vi "Dense - Scale Problem Linear.vi"(8 "error in (no error)":errorcluster, 9 "Y Scaling limits":cluster{"Y lower":dbl, "Y upper":dbl}={"Y lower"=nan, "Y upper"=nan}, 10 "X Scaling limits":cluster{"X lower":dbl, "X upper":dbl}={"X lower"=0.0, "X upper"=1.0}, 11 "Problem":T1) -> (0 "error out":errorcluster, 1 "ymaxmin":cluster{"ymax":dbl, "ymin":dbl}, 2 "xmaxmin":cluster{"min":dbl, "max":dbl}[](array[cluster]), 3 "Scaled problem":T1)   [LabVIEW 2015]
doc: "Scales the problem similarly to the svm-scale tool bundled with libsvm.\nAlways use the output from this VI to scale the test set instead of scaling individually.\n\nNote that dense and sparse xmaxmin are not compatible, as the 0th index is unused for sparse."
uses:
  LibSVM Dense/Wrapper API/Controls/svmdense_problem.ctl
  Controls/Statemachine_ScaleProblem.ctl
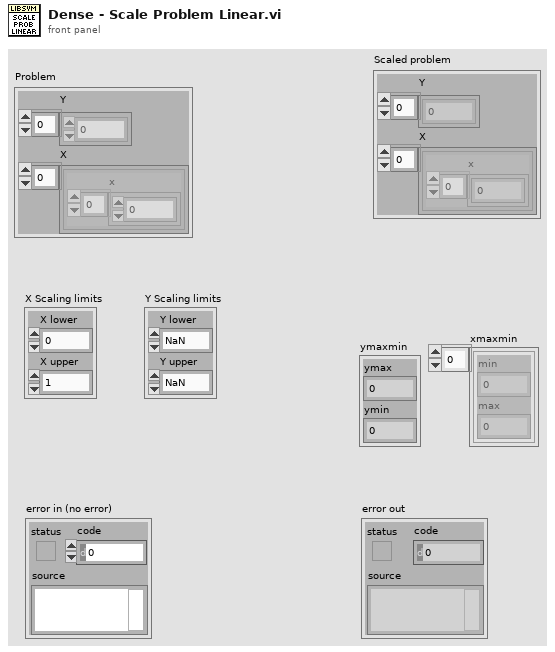
[diagram p1: front panel]
types:
  T1 = typedef "svmdense_problem.ctl" = cluster{"Y":dbl[], "X":cluster{"x":dbl[]}[]}
  T2 = typedef "Statemachine_ScaleProblem.ctl" = enum16{"Input verification: Limits", "Input verification: Ascending indices", "Find max/min index", "Find max/min features", "Scale", "Stop"}
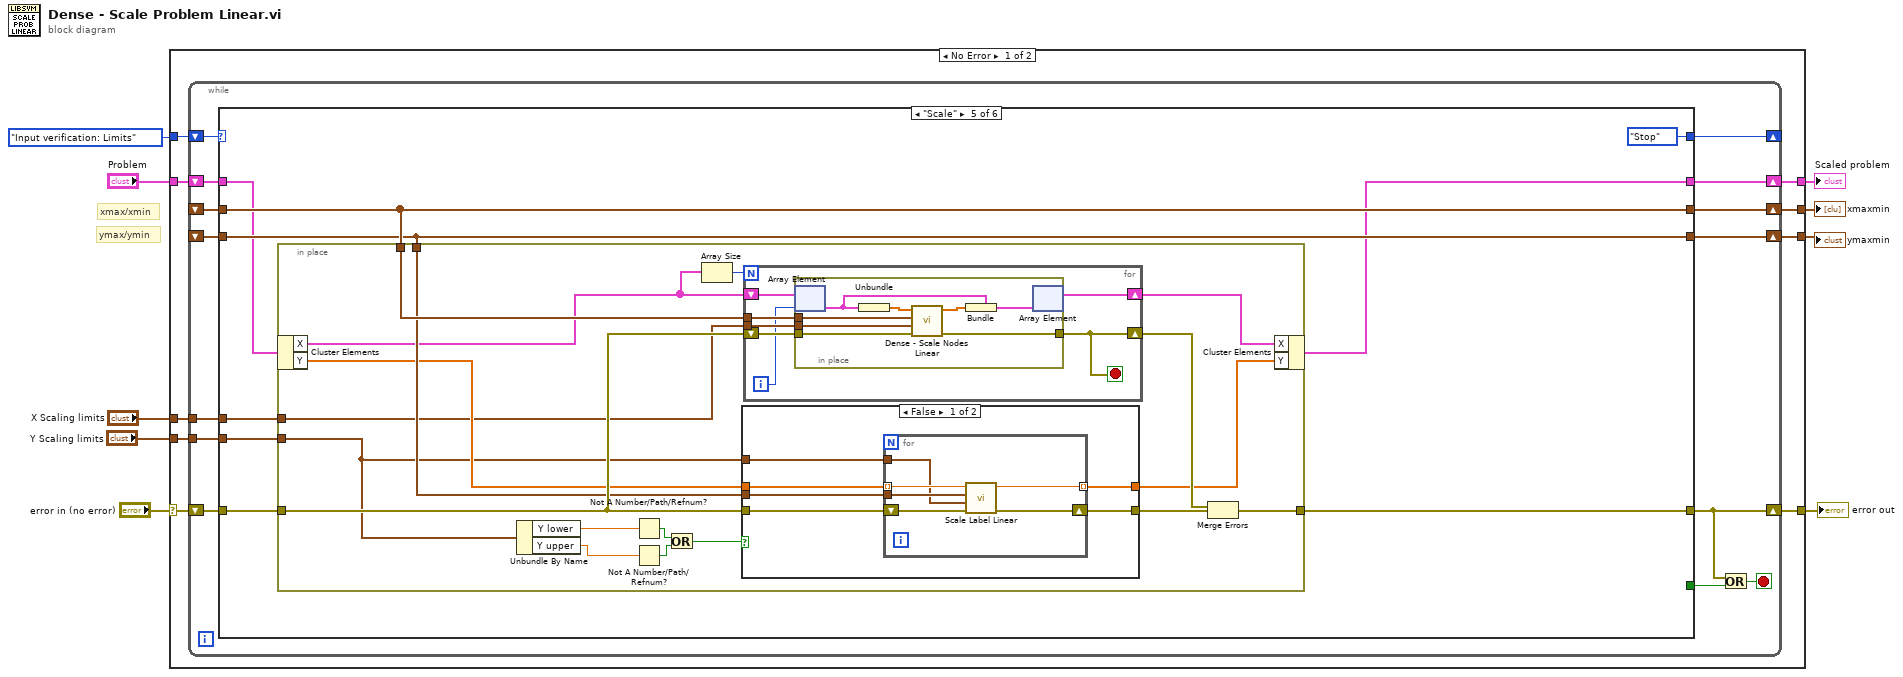
[diagram p0: block diagram]
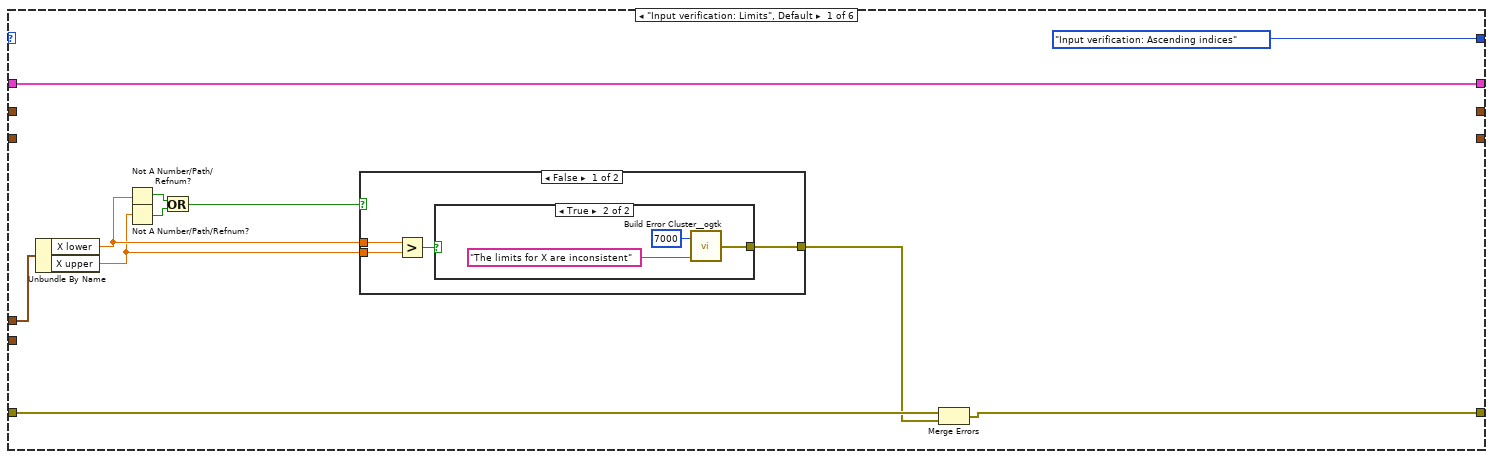
[diagram p2: hidden frame]
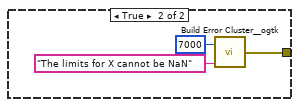
[diagram p4: hidden frame]
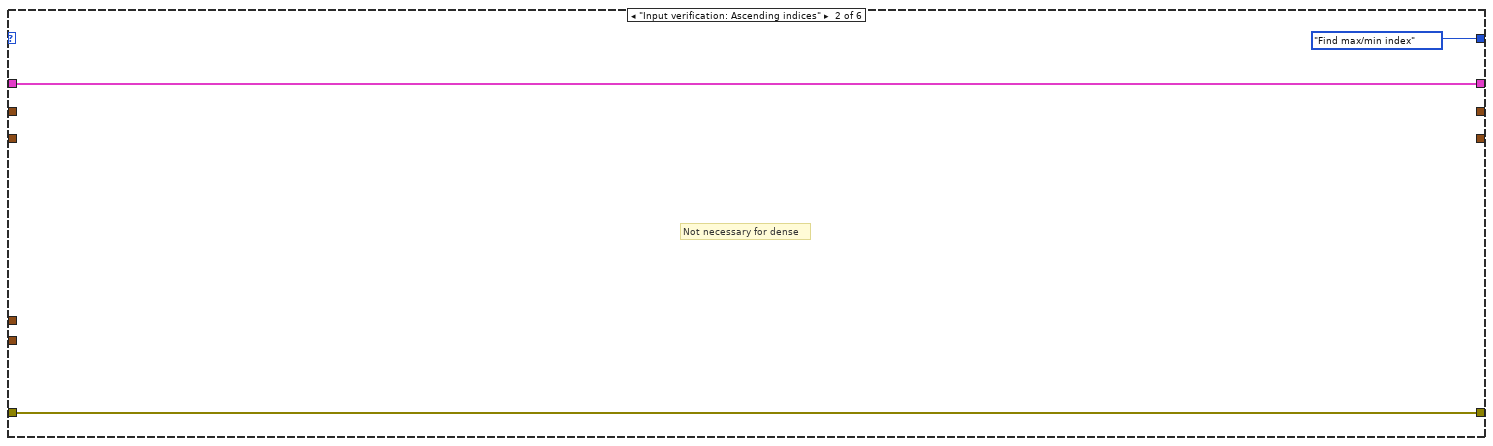
[diagram p5: hidden frame]
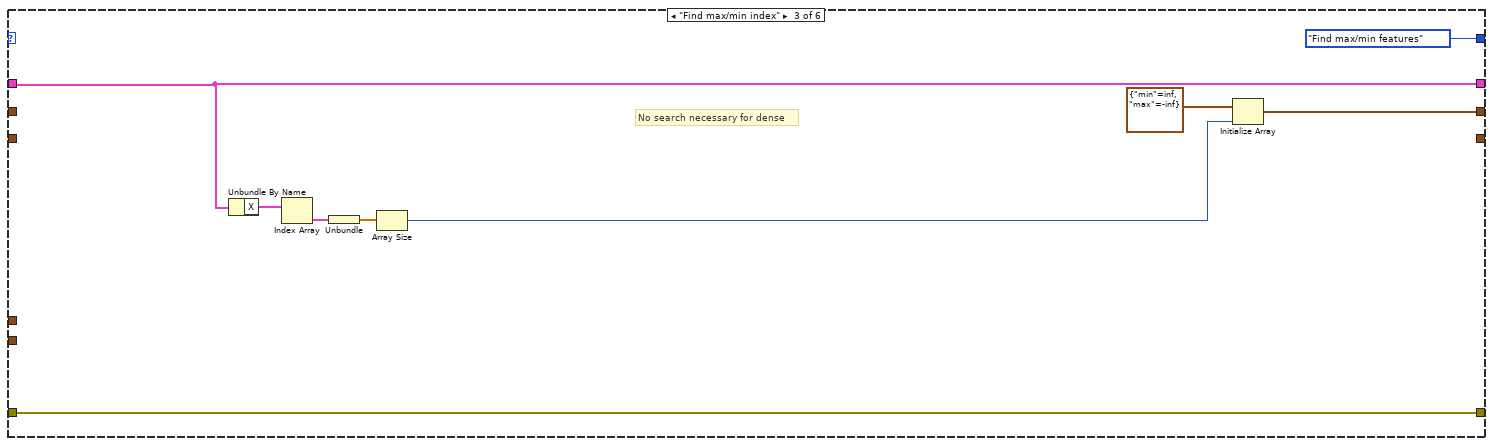
[diagram p6: hidden frame]
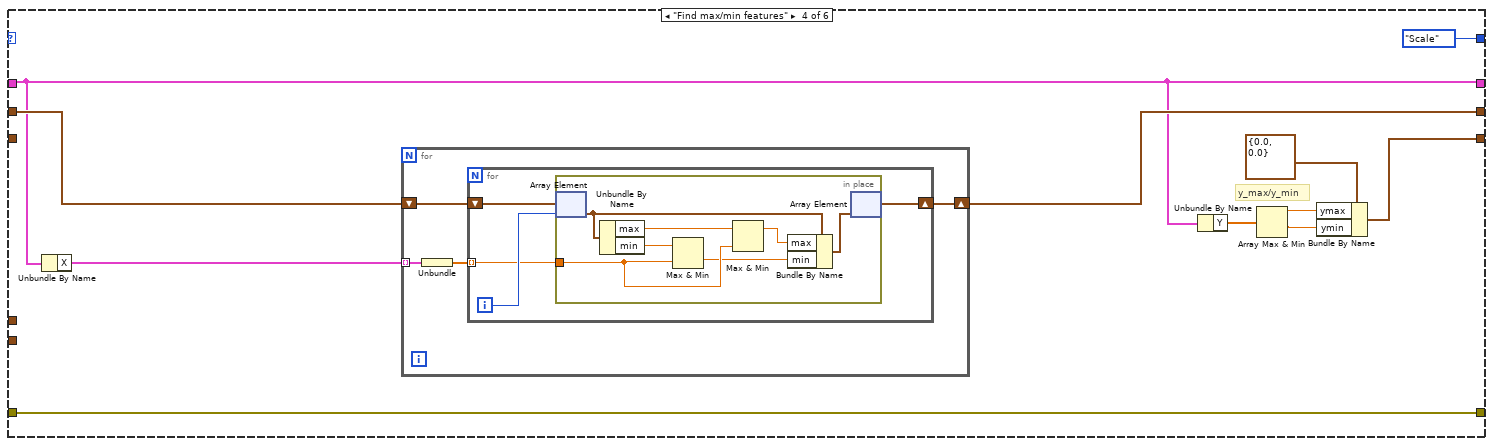
[diagram p7: hidden frame]
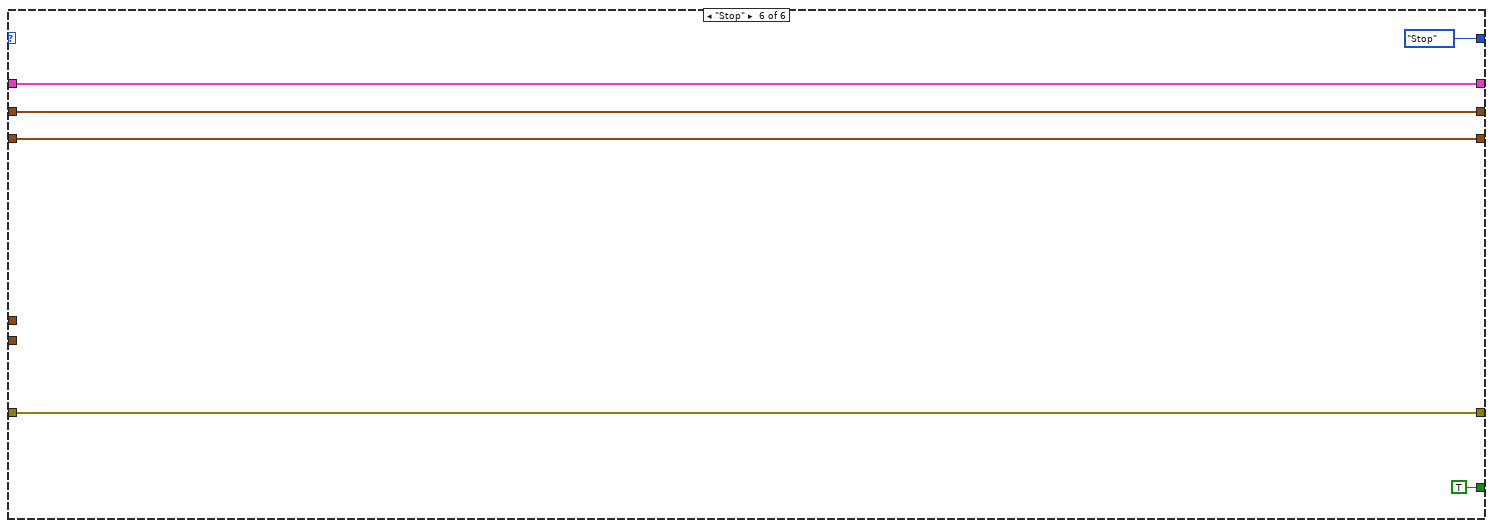
[diagram p9: hidden frame]
diagram:
  # "ymax/ymin"
  # "xmax/xmin"
  n1 = case shown="No Error" "error in (no error)" {
    selector: "error in (no error)" -> [w18 w154]
    tunnel: [w15 w154] -> w9
    tunnel: "Problem" -> [w11 _]
    tunnel: "X Scaling limits" -> [w16 _]
    tunnel: Statemachine_ScaleProblem."Input verification: Limits" ("Statemachine_ScaleProblem") -> [w17 _]
    tunnel: [w14 _] -> w4
    tunnel: [w13 _] -> w5
    tunnel: [w12 _] -> w2
    tunnel: "Y Scaling limits" -> [w10 _]
    frame No Error {
      n2 = while {
        shift-right: [w29] -> _
        shift-left: w17 -> [w32]
        tunnel: w16 -> [w31]
        shift-right: [w22] -> w15
        shift-left: w18 -> [w30]
        shift-right: [w28] -> w13
        shift-left: _ -> [w27]
        shift-right: [w26] -> w14
        shift-left: _ -> [w25]
        shift-right: [w24] -> w12
        shift-left: w11 -> [w23]
        tunnel: w10 -> [w19]
        stop <- w21 stop-if-true
        n3 = case shown="\"Scale\"" w32 {
          tunnel: w31 -> [w43 _ _ _ w99 _]
          tunnel: w30 -> [w37 w56 w57 w73 w98 w152]
          tunnel: [w35 w56 w57 w73 w97 w152] -> w22
          tunnel: [Statemachine_ScaleProblem."Input verification: Ascending indices" ("Statemachine_ScaleProblem") Statemachine_ScaleProblem."Find max/min index" ("Statemachine_ScaleProblem") Statemachine_ScaleProblem."Find max/min features" ("Statemachine_ScaleProblem") Statemachine_ScaleProblem."Scale" ("Statemachine_ScaleProblem") Statemachine_ScaleProblem."Stop" ("Statemachine_ScaleProblem") Statemachine_ScaleProblem."Stop" ("Statemachine_ScaleProblem")] -> w29
          tunnel: [_ _ w64 w74 w96 w151] -> w28
          tunnel: w27 -> [_ _ _ w75 w96 w151]
          tunnel: [_ _ _ w69 w95 w150] -> w26
          tunnel: w25 -> [_ _ _ _ w95 w150]
          tunnel: [w33 w54 w62 w67 w93 w149] -> w24
          tunnel: w23 -> [w33 w54 w62 w67 w94 w149]
          tunnel: [_ _ _ _ _ TRUE] -> w20
          tunnel: w19 -> [_ _ _ _ w92 _]
          frame "Input verification: Limits", Default {
            n4 = Unbundle By Name(w43) -> ("X lower"=w39:dbl, "X upper"=w38:dbl)
            n5 = Not A Number/Path/Refnum?(number/path/refnum=w39) -> (NaN/Path/Refnum?=w41:bool)
            n6 = Not A Number/Path/Refnum?(number/path/refnum=w38) -> (NaN/Path/Refnum?=w42:bool)
            n7 = Or(x=w41, y=w42) -> (x .or. y?=w40:bool)
            n8 = case shown="False" w40 {
              tunnel: w39 -> [w46 _]
              tunnel: w38 -> [w45 _]
              tunnel: [w44 w51] -> w36
              frame False {
                n9 = Greater?(x=w46, y=w45) -> (0:w47:bool)
                n10 = case shown="True" w47 {
                  tunnel: [_ w48] -> w44
                  frame False {
                  }
                  frame True {
                    n11 = call <userlib>:"Build Error Cluster__ogtk.vi"("String to Prepend to source (\"\")"="The limits for X are inconsistent" ("String to Prepend to source (\"\")"), "code"=7000) -> ("error out"=w48:errorcluster)
                  }
                }
              }
              frame True {
                n12 = call <userlib>:"Build Error Cluster__ogtk.vi"("String to Prepend to source (\"\")"="The limits for X cannot be NaN" ("String to Prepend to source (\"\")"), "code"=7000) -> ("error out"=w51:errorcluster)
              }
            }
            n13 = Merge Errors(w37, w36) -> (w35:errorcluster)
          }
          frame "Input verification: Ascending indices" {
            # "Not necessary for dense"
          }
          frame "Find max/min index" {
            # "No search necessary for dense"
            n14 = Unbundle By Name(w62) -> ("X"=w61:cluster{"x":dbl[]}[])
            n15 = Index Array(array=w61) -> (element=w60:cluster{"x":dbl[]})  [unwired: 1 in]
            n16 = Unbundle(w60) -> ("x"=w59:dbl[])
            n17 = Array Size(array=w59) -> (size(s)=w58:i32)
            n18 = Initialize Array(cluster{"min":dbl, "max":dbl} {"min"=inf, "max"=-inf}, w58) -> (w64:cluster{"min":dbl, "max":dbl}[])
          }
          frame "Find max/min features" {
            # "y_max/y_min"
            n19 = Unbundle By Name(w67) -> ("X"=w76:cluster{"x":dbl[]}[])
            n20 = for {
              tunnel: w76 -> [w80] mode=indexing
              shift-right: [w78] -> w74
              shift-left: w75 -> [w79]
              n21 = Unbundle(w80) -> ("x"=w77:dbl[])
              n22 = for {
                shift-right: [w83] -> w78
                shift-left: w79 -> [w84]
                tunnel: w77 -> [w81] mode=indexing
                i -> [w82]
                n23 = in-place {
                  in-place-border: w81 -> [w89]
                  n24 = in-place-array #1(w84, w82) -> (w88:cluster{"min":dbl, "max":dbl})
                  n25 = Unbundle By Name(w88) -> ("max"=w90:dbl, "min"=w91:dbl)
                  n26 = Max & Min(x=w91, y=w89) -> (min(x,y)=w86:dbl)  [unwired: 1 out]
                  n27 = Max & Min(x=w90, y=w89) -> (max(x,y)=w85:dbl)  [unwired: 1 out]
                  n28 = Bundle By Name(cluster=w88, "max"=w85, "min"=w86) -> (w87:cluster{"min":dbl, "max":dbl})
                  n29 = in-place-array #1(w87) -> (w83:cluster{"min":dbl, "max":dbl}[])  [unwired: 1 out]
                }
              }
            }
            n30 = Unbundle By Name(w67) -> ("Y"=w66:dbl[])
            n31 = Array Max & Min(array=w66) -> (max value=w71:dbl, min value=w70:dbl)  [unwired: 2 out]
            n32 = Bundle By Name(cluster=cluster{"ymax":dbl, "ymin":dbl} {"ymax"=0.0, "ymin"=0.0}, "ymax"=w71, "ymin"=w70) -> (w69:cluster{"ymax":dbl, "ymin":dbl})
          }
          frame "Scale" {
            n33 = in-place {
              in-place-border: w99 -> [w104]
              in-place-border: w98 -> [w118]
              in-place-border: [w117] -> w97
              in-place-border: w96 -> [w111]
              in-place-border: w95 -> [w110]
              in-place-border: w92 -> [w101]
              n34 = in-place-cluster #2(w94) -> ("X"=w106:cluster{"x":dbl[]}[], "Y"=w109:dbl[])
              n35 = Unbundle By Name(w101) -> ("Y lower"=w103:dbl, "Y upper"=w102:dbl)
              n36 = Not A Number/Path/Refnum?(number/path/refnum=w103) -> (NaN/Path/Refnum?=w114:bool)
              n37 = Not A Number/Path/Refnum?(number/path/refnum=w102) -> (NaN/Path/Refnum?=w113:bool)
              n38 = Or(x=w114, y=w113) -> (x .or. y?=w112:bool)
              n39 = Array Size(array=w106) -> (size(s)=w107:i32)
              n40 = case shown="False" w112 {
                tunnel: w118 -> [w124 w131]
                tunnel: w109 -> [w123 w132]
                tunnel: w110 -> [w122 _]
                tunnel: [w121 w131] -> w116
                tunnel: [w120 w132] -> w108
                tunnel: w101 -> [w119 _]
                frame False {
                  n41 = for {
                    shift-right: [w129] -> w121
                    shift-left: w124 -> [w130]
                    tunnel: w123 -> [w128] mode=indexing
                    tunnel: w119 -> [w125]
                    tunnel: w122 -> [w127]
                    tunnel: [w126] -> w120 mode=indexing
                    n42 = call "Scale Label Linear.vi"("error in (no error)"=w130, "Scaling limits"=w125, "ymaxmin"=w127, "y"=w128) -> ("error out"=w129:errorcluster, "y scaled"=w126:dbl)  [unwired: 6 in]
                  }
                }
                frame True {
                  # "NaN y limit - do not perform scaling"
                }
              }
              n43 = for {
                N: w107 -> [_]
                tunnel: w111 -> [w138]
                shift-right: [w133] -> w115
                shift-left: w118 -> [w139]
                tunnel: w104 -> [w137]
                shift-right: [w134] -> w105
                shift-left: w106 -> [w136]
                i -> [w135]
                stop <- w133 stop-if-true
                n44 = in-place {
                  in-place-border: w139 -> [w144]
                  in-place-border: w138 -> [w141]
                  in-place-border: [w143] -> w133
                  in-place-border: w137 -> [w140]
                  n45 = in-place-array #3(w136, w135) -> (w146:cluster{"x":dbl[]})
                  n46 = Unbundle(w146) -> ("x"=w142:dbl[])
                  n47 = call "Dense - Scale Nodes Linear.vi"("error in (no error)"=w144, "Scaling limits"=w140, "xmaxmin"=w141, "x"=w142) -> ("error out"=w143:errorcluster, "x scaled"=w145:dbl[])  [unwired: 6 in]
                  n48 = Bundle(cluster=w146, "x"=w145) -> (w147:cluster{"x":dbl[]})
                  n49 = in-place-array #3(w147) -> (w134:cluster{"x":dbl[]}[])  [unwired: 1 out]
                }
              }
              n50 = Merge Errors(w115, w116) -> (w117:errorcluster)
              n51 = in-place-cluster #2("X"=w105, "Y"=w108) -> (w93:T1)
            }
          }
          frame "Stop" {
          }
        }
        n52 = Or(x=w22, y=w20) -> (x .or. y?=w21:bool)
      }
    }
    frame Error {
    }
  }
  "error out" <- w9
  "xmaxmin" <- w5
  "ymaxmin" <- w4
  "Scaled problem" <- w2
